vi "MoveBaseAbs.vi"(8 "error in (no error)":errorcluster caption="Fehler (Eingang, kein Fehler)", 9 "Speed":i16=120, 10 "Base":dbl, 11 "Moveo Eingang":refnum<class "Moveo.lvclass">) -> (0 "error out":errorcluster caption="Fehler (Ausgang)", 3 "Moveo Ausgang":refnum<class "Moveo.lvclass">)   [LabVIEW 2019, in "Moveo.lvclass"]
uses:
  Moveo.lvclass
  Moveo.lvclass/Moveo.ctl
  MoveoSerialClass/MoveoSerial.lvclass
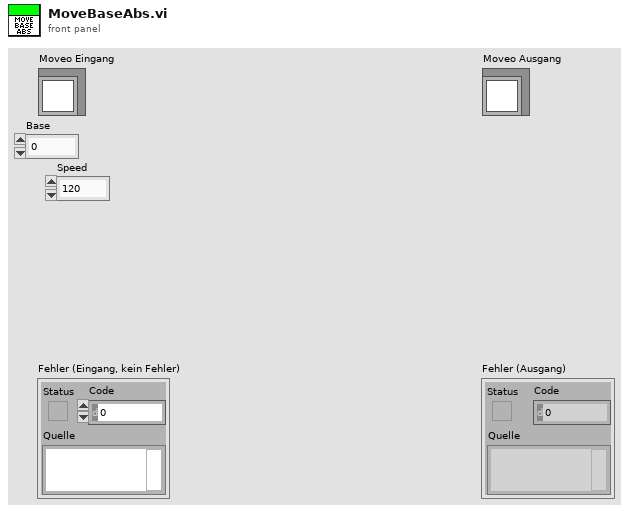
[diagram p1: front panel]
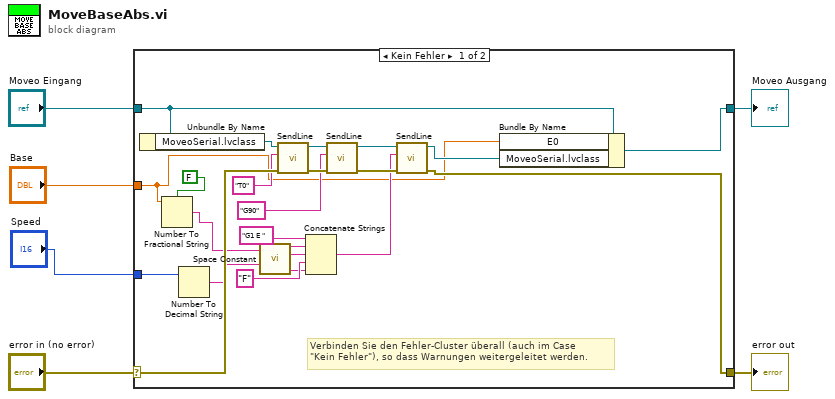
[diagram p0: block diagram]
diagram:
  n1 = case shown="Kein Fehler" "error in (no error)" {
    selector: "error in (no error)" -> [w26 w29]
    tunnel: [w10 w29] -> w5
    tunnel: [w12 w28] -> w3
    tunnel: "Moveo Eingang" -> [w13 w28]
    tunnel: "Base" -> [w9 _]
    tunnel: "Speed" -> [w19 _]
    frame No Error {
      # "Verbinden Sie den Fehler-Cluster überall (auch im Case\n\"Kein Fehler\"), so dass Warnungen weitergeleitet werden."
      n2 = Unbundle By Name(w13) -> ("MoveoSerial.lvclass"=w27:refnum<class "MoveoSerial.lvclass">)
      n3 = Number To Fractional String(use system decimal point (T)=FALSE, number=w9) -> (F-format string=w8:string)  [unwired: 2 in]
      n4 = Number To Decimal String(number=w19) -> (decimal integer string=w17:string)  [unwired: 1 in]
      n5 = call <vilib>:"Space Constant.vi"() -> ("String"=w20:string)
      n6 = call-dynamic "SendLine.vi"("error in (no error)"=w26, "SendString"="T0", "MoveoSerial Eingang"=w27) -> ("error out"=w24:errorcluster, "MoveoSerial Ausgang"=w23:refnum<class "MoveoSerial.lvclass">)  [unwired: 7 in]
      n7 = Concatenate Strings("G1 E ", w8, w20, "F", w17) -> (w14:string)
      n8 = call-dynamic "SendLine.vi"("error in (no error)"=w24, "SendString"="G90", "MoveoSerial Eingang"=w23) -> ("error out"=w15:errorcluster, "MoveoSerial Ausgang"=w16:refnum<class "MoveoSerial.lvclass">)  [unwired: 7 in]
      n9 = call-dynamic "SendLine.vi"("error in (no error)"=w15, "SendString"=w14, "MoveoSerial Eingang"=w16) -> ("error out"=w10:errorcluster, "MoveoSerial Ausgang"=w11:refnum<class "MoveoSerial.lvclass">)  [unwired: 7 in]
      n10 = Bundle By Name(cluster=w13, "E0"=w9, "MoveoSerial.lvclass"=w11) -> (w12:refnum<class "Moveo.lvclass">)
    }
    frame Error {
    }
  }
  "error out" <- w5
  "Moveo Ausgang" <- w3
